vi "HEWH Check UE Cutout For Condition Change.vi"(6 "End of Draw Comparison":bool[][](array[boolean]), 7 "HEWH Specific DAQ":T8, 9 "Current Sequence Index":i32, 10 "Current Sequence":T1={"Sequence #"=0.0, "Cycles"=0, "Mode Setting"="", "Flow Rate (GPM)"=0.0, "Temperature (F)"=0.0, "Reset Timer"=FALSE, "Use Temp Decline Method"=FALSE, "Terminate Condition"=enum."C1-Terminate Draw @ Gallon Mark", "Condition Value #1"=0.0, "UE"=FALSE, "LE"=FALSE, "Comp"=FALSE, "Fan"=FALSE, "Test End Time (Sec)"=0.0, "Purge Until Cutout"=FALSE, "Start Conditions"=enum."Heat Source Cutout", "Condition Value #2"=0.0, "Remove Power"=FALSE, "Time"=0.0, "Check Special Cond."=enum."SC1-Do Nothing", "Condition#"=enum."C1", "Draw Flags"=enum."N/A", "Data Processing Delay (FHD 15sec, UEF 5 Sec)"=0.0, "Test Complete"=FALSE, "User Setpoint"=0.0, "Tank Setpoint"=0.0} {"Time" format="%<%H:%M:%S>t"}, 11 "PRAT/RLT Sequence":T1[](array[typedef]) {"Time" format="%<%H:%M:%S>t"}) -> (2 "Terminate Condition out":T3, 3 "PRAT/RLT Sequence (Output)":T1[](array[typedef]) {"Time" format="%<%H:%M:%S>t"}, 4 "End of Draw Comparison Output":bool[][](array[boolean]))   [LabVIEW 2019]
uses:
  Type Definitions/HEWH Specific DAQ.ctl
  Type Definitions/HEWH Power Data.ctl
  Type Definitions/HEWH Power Elements.ctl
  Utility/Type Definitions/UTILITY Power Analyzer.ctl
  Draw Water Specific/Type Definitions/Terminate Draw Conditions.ctl
  Type Definitions/PRAT Test.ctl
  Utility/Save File/File Setup (Public)/Type Definition/Save File HEWH Heating Control Mode.ctl
  Type Definitions/HEWH Start Conditions.ctl
  Draw Water Specific/Type Definitions/Check Special Condtions.ctl
  Draw Water Specific/Type Definitions/HEWH Special Condition Check.ctl
  Type Definitions/HEWH Draw Flag ENUM.ctl
  Utility/Type Definitions/UTILITY Notifier.ctl
  Utility/Save File/File Setup.lvlib
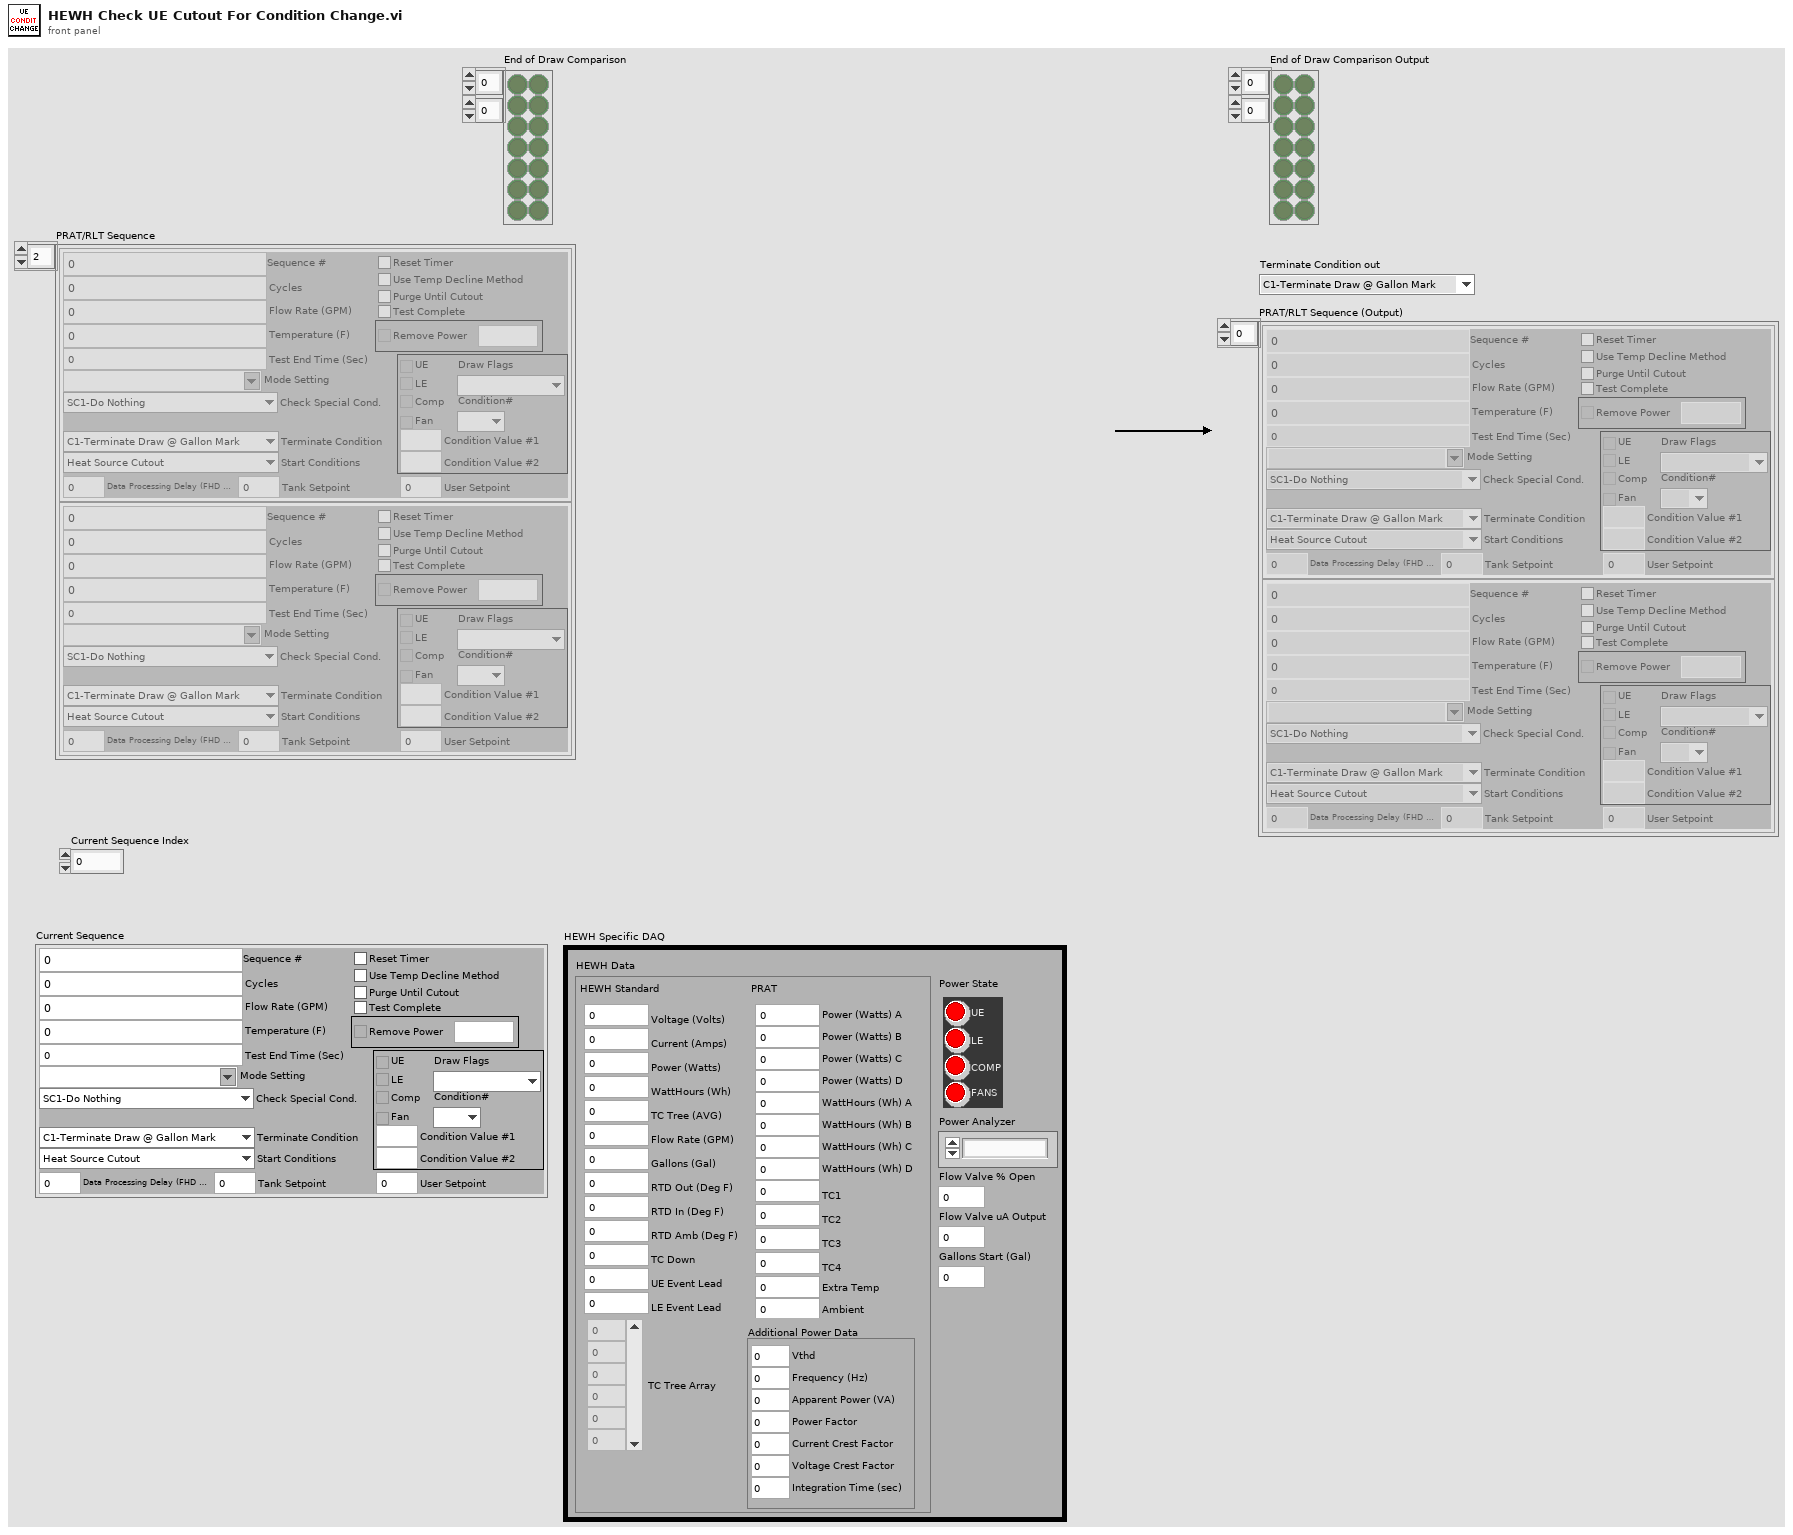
[diagram p1: front panel]
types:
  T1 = typedef "PRAT Test.ctl" = cluster{"Sequence #":dbl, "Cycles":i32, "Mode Setting":T2, "Flow Rate (GPM)":dbl, "Temperature (F)":dbl, "Reset Timer":bool, "Use Temp Decline Method":bool, "Terminate Condition":T3, "Condition Value #1":dbl, "UE":bool, "LE":bool, "Comp":bool, "Fan":bool, "Test End Time (Sec)":dbl, "Purge Until Cutout":bool, "Start Conditions":T4, "Condition Value #2":dbl, "Remove Power":bool, "Time":dbl, "Check Special Cond.":T5, "Condition#":T6, "Draw Flags":T7, "Data Processing Delay (FHD 15sec, UEF 5 Sec)":dbl, "Test Complete":bool, "User Setpoint":dbl, "Tank Setpoint":dbl}
  T2 = typedef "File Setup.lvlib/Save File HEWH Heating Control Mode.ctl" = string
  T3 = typedef "Terminate Draw Conditions.ctl" = enum16{"C1-Terminate Draw @ Gallon Mark", "C2-Special Last Draw (HU Test)", "C3-RTD Out <=", "C4-Mean Tank Temp <=", "C5-Decrease RTD Out (Deg F)", "C6-Time (Seconds)", "C7-Until Any Heat Source", "C8-Specific Heat Source", "C9-Do Nothing", "C10-Inlet Outlet RTD Temp Delta"}
  T4 = typedef "HEWH Start Conditions.ctl" = enum16{"Heat Source Cutout", "At Time (Seconds)", "Every X (Seconds)", "T2 >= X° Below Setpoint", "Seconds From Complete", "Wait for LE & Comp Cutout", "Wait for Comp Cutout", "Wait for LE Cutout", "Wait for UE Cutout", "Start Immediately"}
  T5 = typedef "Check Special Condtions.ctl" = enum16{"SC1-Do Nothing", "SC2-Check Heat Source (On-C2/Off-C1)", "SC3-Check Skip Condition", "SC4-Check Heat Source ON/Fail", "SC5-Keep Draw Valves Open", "SC6-Skip Purge"}
  T6 = typedef "HEWH Special Condition Check.ctl" = enum16{"N/A", "C1", "C2", "Reset/Fail", "Skip Draw Sequence"}
  T7 = typedef "HEWH Draw Flag ENUM.ctl" = enum16{"N/A", "None(0)", "Sml(1)", "Med(2)", "SmlMed(3)", "Lrg(4)", "SmlLrg(5)", "MedLrg(6)", "SmlMedLrg(7)"}
  T8 = typedef "HEWH Specific DAQ.ctl" = cluster{"HEWH Data":T9, "Flow Valve % Open":dbl, "Power State":T10, "Power Analyzer":T11, "Flow Valve uA Output":i32, "Gallons Start (Gal)":dbl}
  T9 = typedef "HEWH Power Data.ctl" = cluster{"HEWH Standard":cluster{"Voltage (Volts)":dbl, "Current (Amps)":dbl, "Power (Watts)":dbl, "WattHours (Wh)":dbl, "TC Tree (AVG)":dbl, "Flow Rate (GPM)":dbl, "Gallons (Gal)":dbl, "RTD Out (Deg F)":dbl, "RTD In (Deg F)":dbl, "RTD Amb (Deg F)":dbl, "TC Down":dbl, "UE Event Lead":i32, "LE Event Lead":i32, "TC Tree Array":dbl[]}, "PRAT":cluster{"Power (Watts) A":dbl, "Power (Watts) B":dbl, "Power (Watts) C":dbl, "Power (Watts) D":dbl, "TC1":dbl, "TC2":dbl, "TC3":dbl, "TC4":dbl, "WattHours (Wh) A":dbl, "WattHours (Wh) B":dbl, "WattHours (Wh) C":dbl, "WattHours (Wh) D":dbl, "Ambient":dbl, "Extra Temp":dbl}, "Additional Power Data":cluster{"Vthd":dbl, "Frequency (Hz)":dbl, "Apparent Power (VA)":dbl, "Power Factor":dbl, "Current Crest Factor":dbl, "Voltage Crest Factor":dbl, "Integration Time (sec)":dbl}}
  T10 = typedef "HEWH Power Elements.ctl" = cluster{"UE":bool, "LE":bool, "COMP":bool, "FANS":bool}
  T11 = typedef "UTILITY Power Analyzer.ctl" = enum16{"", "APLUS", "WT210", "WT500", "WT300", "OSI", "Debug", "WT230", "WT300_1", "WT300_2"}
  T12 = typedef "UTILITY Notifier.ctl" = enum16{"Set", "Read", "Release Ref"}
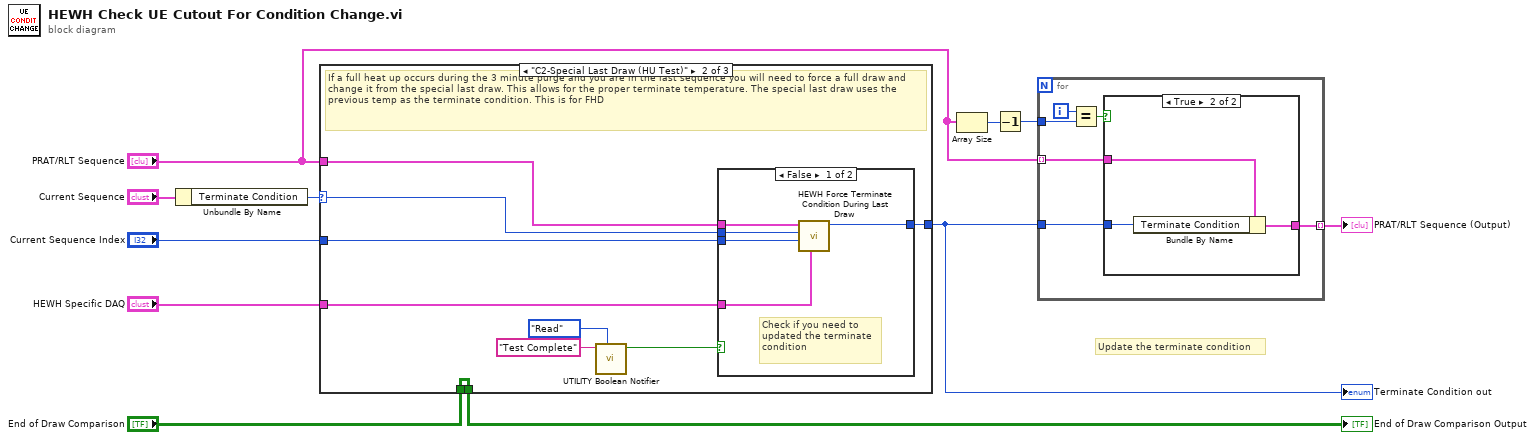
[diagram p0: block diagram]
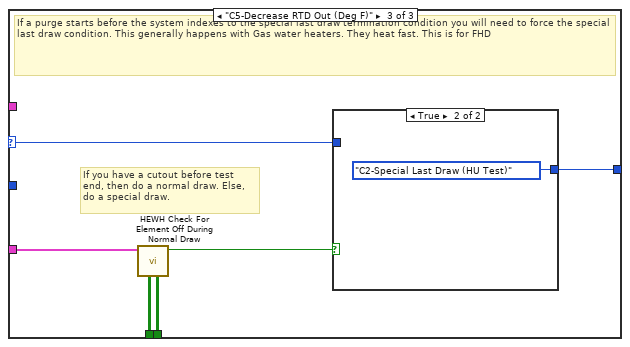
[diagram p4: hidden frame]
diagram:
  # "Update the terminate condition"
  n1 = Unbundle By Name("Current Sequence") -> ("Terminate Condition"=w7:T3)
  n2 = case shown="\"C2-Special Last Draw (HU Test)\"" w7 {
    selector: w7 -> [w13 w20 w33]
    tunnel: "HEWH Specific DAQ" -> [_ w22 w31]
    tunnel: "Current Sequence Index" -> [_ w21 _]
    tunnel: "PRAT/RLT Sequence" -> [_ w19 _]
    tunnel: [w13 w18 w32] -> w3
    tunnel: "End of Draw Comparison" -> [w12 w14 w30]
    tunnel: [w12 w14 w29] -> w1
    frame Default {
    }
    frame "C2-Special Last Draw (HU Test)" {
      # "If a full heat up occurs during the 3 minute purge and you are in the last sequence you will need to force a full draw and change it from the special last draw. This allows for the proper terminate temperature. The special last draw uses the previous temp as the terminate condition. This is for FHD"
      n3 = call "UTILITY Boolean Notifier.vi"("Status"=UTILITY_Notifier."Read", "name (unnamed)"="Test Complete") -> ("latest READ notification"=w15:bool)  [unwired: 8 in, 1 out]
      n4 = case shown="False" w15 {
        tunnel: w22 -> [w27 _]
        tunnel: w21 -> [w26 _]
        tunnel: w20 -> [w25 w28]
        tunnel: w19 -> [w24 _]
        tunnel: [w23 w28] -> w18
        frame False {
          # "Check if you need to\nupdated the terminate\ncondition"
          n5 = call "HEWH Force Terminate Condition During Last Draw.vi"("HEWH Specific DAQ"=w27, "Current Sequence Index"=w26, "Terminate Condition in"=w25, "PRAT/RLT Sequence"=w24) -> ("Terminate Condition out"=w23:T3)  [unwired: 7 in]
        }
        frame True {
          # "No more changes\nafter test complete"
        }
      }
    }
    frame "C5-Decrease RTD Out (Deg F)" {
      # "If you have a cutout before test\nend, then do a normal draw. Else,\ndo a special draw."
      # "If a purge starts before the system indexes to the special last draw termination condition you will need to force the special last draw condition. This generally happens with Gas water heaters. They heat fast. This is for FHD"
      n6 = call "HEWH Check For Element Off During Normal Draw.vi"("End of Draw Comparison"=w30, "HEWH Specific DAQ"=w31) -> ("Cutout after Test Complete"=w34:bool, "End of Draw Comparison Output"=w29:bool[][])  [unwired: 8 in]
      n7 = case shown="True" w34 {
        tunnel: w33 -> [w35 _]
        tunnel: [w35 Terminate_Draw_Conditions."C2-Special Last Draw (HU Test)" ("Terminate Condition")] -> w32
        frame False {
        }
        frame True {
        }
      }
    }
  }
  "Terminate Condition out" <- w3
  "End of Draw Comparison Output" <- w1
  n8 = Array Size(array="PRAT/RLT Sequence") -> (size(s)=w11:i32)
  n9 = Decrement(x=w11) -> (x-1=w10:i32)
  n10 = for {
    tunnel: "PRAT/RLT Sequence" -> [w39] mode=indexing
    tunnel: w10 -> [w42]
    tunnel: [w38] -> w9 mode=indexing
    tunnel: w3 -> [w37]
    i -> [w41]
    n11 = Equal?(x=w41, y=w42) -> (x = y?=w40:bool)
    n12 = case shown="True" w40 {
      tunnel: w39 -> [w43 w46]
      tunnel: [w43 w45] -> w38
      tunnel: w37 -> [_ w44]
      frame False {
      }
      frame True {
        n13 = Bundle By Name(cluster=w46, "Terminate Condition"=w44) -> (w45:T1)
      }
    }
  }
  "PRAT/RLT Sequence (Output)" <- w9
